vi "Dual_PID_tester.vi"() -> ()   [LabVIEW 2013]
uses:
  DataMode.ctl
  Input_5782/5782_states.ctl
  <vilib>/Platform/TimedLoop/XDataNode/timing_clust.ctl
  <vilib>/Platform/TimedLoop/XDataNode/nitl_modes.ctl
  <vilib>/Platform/TimedLoop/XDataNode/wakeup.ctl
  <vilib>/rvi/FXPMathLib/FxpConvert/subVIs/nifxpmath_Convert_SimConfig.ctl
  <vilib>/fxp/LVFixedPointQuantizationPolicyTypeDef.ctl
  <vilib>/fxp/LVFixedPointOverflowPolicyTypeDef.ctl
  <vilib>/rvi/Emulation/niFpgaSctlEmulationGetInTimedLoop.vi
  <vilib>/rvi/Emulation/niFpgaEmulationReportErrorSimple.vi
  <vilib>/rvi/Emulation/niFpgaGetClockAttributes.vi
  <vilib>/rvi/eio/common/nirviEmuTemplateMethod_errors.vi
  <vilib>/rvi/Emulation/niFpgaCriticalErrorInLSC.vi
  <vilib>/rvi/FXPMathLib/FxpConvert/simVIs/DllFxpConvertTemp_sub.vi
  <vilib>/rvi/FIFO/Fifo_Resource/nirvififoEmulationWriteFpgaImpl.vi
  <vilib>/rvi/DataTransferAndStorage/Container/Common/niFpgaContainerGetUniqueNameForEmu.vi
  <vilib>/rvi/DataTransferAndStorage/Register/Emulation/niFpgaRegisterEmulationFpgaImpl.vi
  <instcachedir>/0/niFpgaRegisterEmulationFpgaImpl_DCF4BC0110594B98B44A971D60CEEC4D.lvgen/niFpgaRegisterEmulationFpgaImpl_DCF4BC0110594B98B44A971D60CEEC4D_011.vi
  <instcachedir>/0/niFpgaRegisterEmulationFpgaImpl_DCF4BC0110594B98B44A971D60CEEC4D.lvgen/niFpgaRegisterEmulationFpgaImpl_DCF4BC0110594B98B44A971D60CEEC4D_012.vi
  <instcachedir>/0/niFpgaRegisterEmulationFpgaImpl_DCF4BC0110594B98B44A971D60CEEC4D.lvgen/niFpgaRegisterEmulationFpgaImpl_DCF4BC0110594B98B44A971D60CEEC4D_003.vi
  <instcachedir>/0/niFpgaRegisterEmulationFpgaImpl_DCF4BC0110594B98B44A971D60CEEC4D.lvgen/niFpgaRegisterEmulationFpgaImpl_DCF4BC0110594B98B44A971D60CEEC4D_007.vi
  <instcachedir>/0/niFpgaRegisterEmulationFpgaImpl_DCF4BC0110594B98B44A971D60CEEC4D.lvgen/niFpgaRegisterEmulationFpgaImpl_DCF4BC0110594B98B44A971D60CEEC4D_008.vi
  <instcachedir>/0/niFpgaRegisterEmulationFpgaImpl_DCF4BC0110594B98B44A971D60CEEC4D.lvgen/niFpgaRegisterEmulationFpgaImpl_DCF4BC0110594B98B44A971D60CEEC4D_021.vi
  <instcachedir>/0/niFpgaRegisterEmulationFpgaImpl_DCF4BC0110594B98B44A971D60CEEC4D.lvgen/niFpgaRegisterEmulationFpgaImpl_DCF4BC0110594B98B44A971D60CEEC4D_020.vi
  <instcachedir>/0/niFpgaRegisterEmulationFpgaImpl_DCF4BC0110594B98B44A971D60CEEC4D.lvgen/niFpgaRegisterEmulationFpgaImpl_DCF4BC0110594B98B44A971D60CEEC4D_009.vi
  <vilib>/rvi/FIFO/Fifo_Resource/nirvififoEmulationReadFpgaImpl.vi
  <vilib>/rvi/interface/RandomDataEmulation/nirviRandomDataMultiElementFPGAFIFO.vi
  <instcachedir>/0/nirviRandomDataMultiElementFPGAFIFO_F2B80EDE0D7944A08478D8D26097D4DB.lvgen/nirviRandomDataMultiElementFPGAFIFO_F2B80EDE0D7944A08478D8D26097D4DB_005.vi
  <vilib>/rvi/interface/RandomDataEmulation/niFpgaRandomDataHandleErrors.vi
  <instcachedir>/0/niFpgaRegisterEmulationFpgaImpl_DCF4BC0110594B98B44A971D60CEEC4D.lvgen/niFpgaRegisterEmulationFpgaImpl_DCF4BC0110594B98B44A971D60CEEC4D_013.vi
  <vilib>/rvi/interface/RandomDataEmulation/nirviRandomDataFPGAFIFO.vi
  <vilib>/Platform/TimedLoop/XDataNode/XDataNode.xnode
  <vilib>/eio/EIONode/EIONode.xnode
  <vilib>/rvi/FXPMathLib/FxpInterpret/XNode/nifxpmath_Interpret.xnode
  <vilib>/rvi/FXPMathLib/FxpConvert/XNode/nifxpmath_Convert.xnode
  <vilib>/rvi/DataTransferAndStorage/Container/XNode/niFpgaContainer.xnode
  <vilib>/rvi/FIFO/Fifo_Resource/nirvififoEmulationWrite.vi
  <vilib>/rvi/FXPMathLib/FxpSub/XNode/nifxpmath_Sub.xnode
  <vilib>/rvi/DataTransferAndStorage/Register/Emulation/niFpgaRegisterEmulation.vi
  <vilib>/rvi/FIFO/Fifo_Resource/nirvififoEmulationRead.vi
  <vilib>/rvi/interface/RandomDataEmulation/nirviRandomDataFpgaMultiElementTemplate.vi
  <vilib>/rvi/interface/RandomDataEmulation/nirviRandomDataFpgaReadWriteTemplate.vi
  <vilib>/Platform/TimedLoop/XDataNode/XDNodeRunTimeDep.lvlib
  <vilib>/rvi/FXPMathLib/sim/FxpSim.dll
panel:
  in  "delay phase":fxp<+,64,64>
  in  "5782 record length":u16=4000 caption="Samples Per Trigger" min=1 step=1
  in  "Trigger Acquisition":bool
  in  "5782 record length":u16=4000 caption="Samples Per Trigger" min=1 step=1
  in  "Trigger Acquisition":bool
  in  "AM phase":fxp<+,64,64>
  in  "Continuous":bool
  in  "Downsample":fxp<+,8,8>=1.0
  in  "new coeffs":bool
  in  "FIR coeffs":fxp<+/-,18,18>[](array[numeric])
  in  "CIC Gain":fxp<+/-,32,1>=0.00390625 format="%#_32g"
  in  "Acquisition running":bool
  in  "Phase output":fxp<+,64,64>[](array[numeric])=[0.0, 0.0, 0.0, 0.0, 0.0, 0.0, 0.0, 0.0]
  in  "Simulated phase 5782":fxp<+,64,64>[](array[numeric])=[0.0, 0.0]
  in  "Mode":T1
  in  "Phase 5782":fxp<+,64,64>[](array[numeric])=[0.0, 0.0]
  out "IO Module\\Trigger Input":bool
  in  "IO Module\\AO Data Sync":bool=TRUE
  in  "IO Module\\SPI Write Data":u16
  out "IO Module\\SPI Read Data":u8
  in  "IO Module\\SPI Read":bool
  in  "IO Module\\SPI Write":bool
  in  "IO Module\\SPI Address":u16
  in  "IO Module\\SPI Device":u8
  out "IO Module\\SPI Idle":bool
  in  "User Command Commit":bool
  in  "User Command":u8
  out "User Command Idle":bool
  out "User Command Status":u8
  in  "User Data 0":u8
  in  "User Data 1":u8
  out "PLL Locked":bool
  out "User Error":bool
  out "Configured?":bool
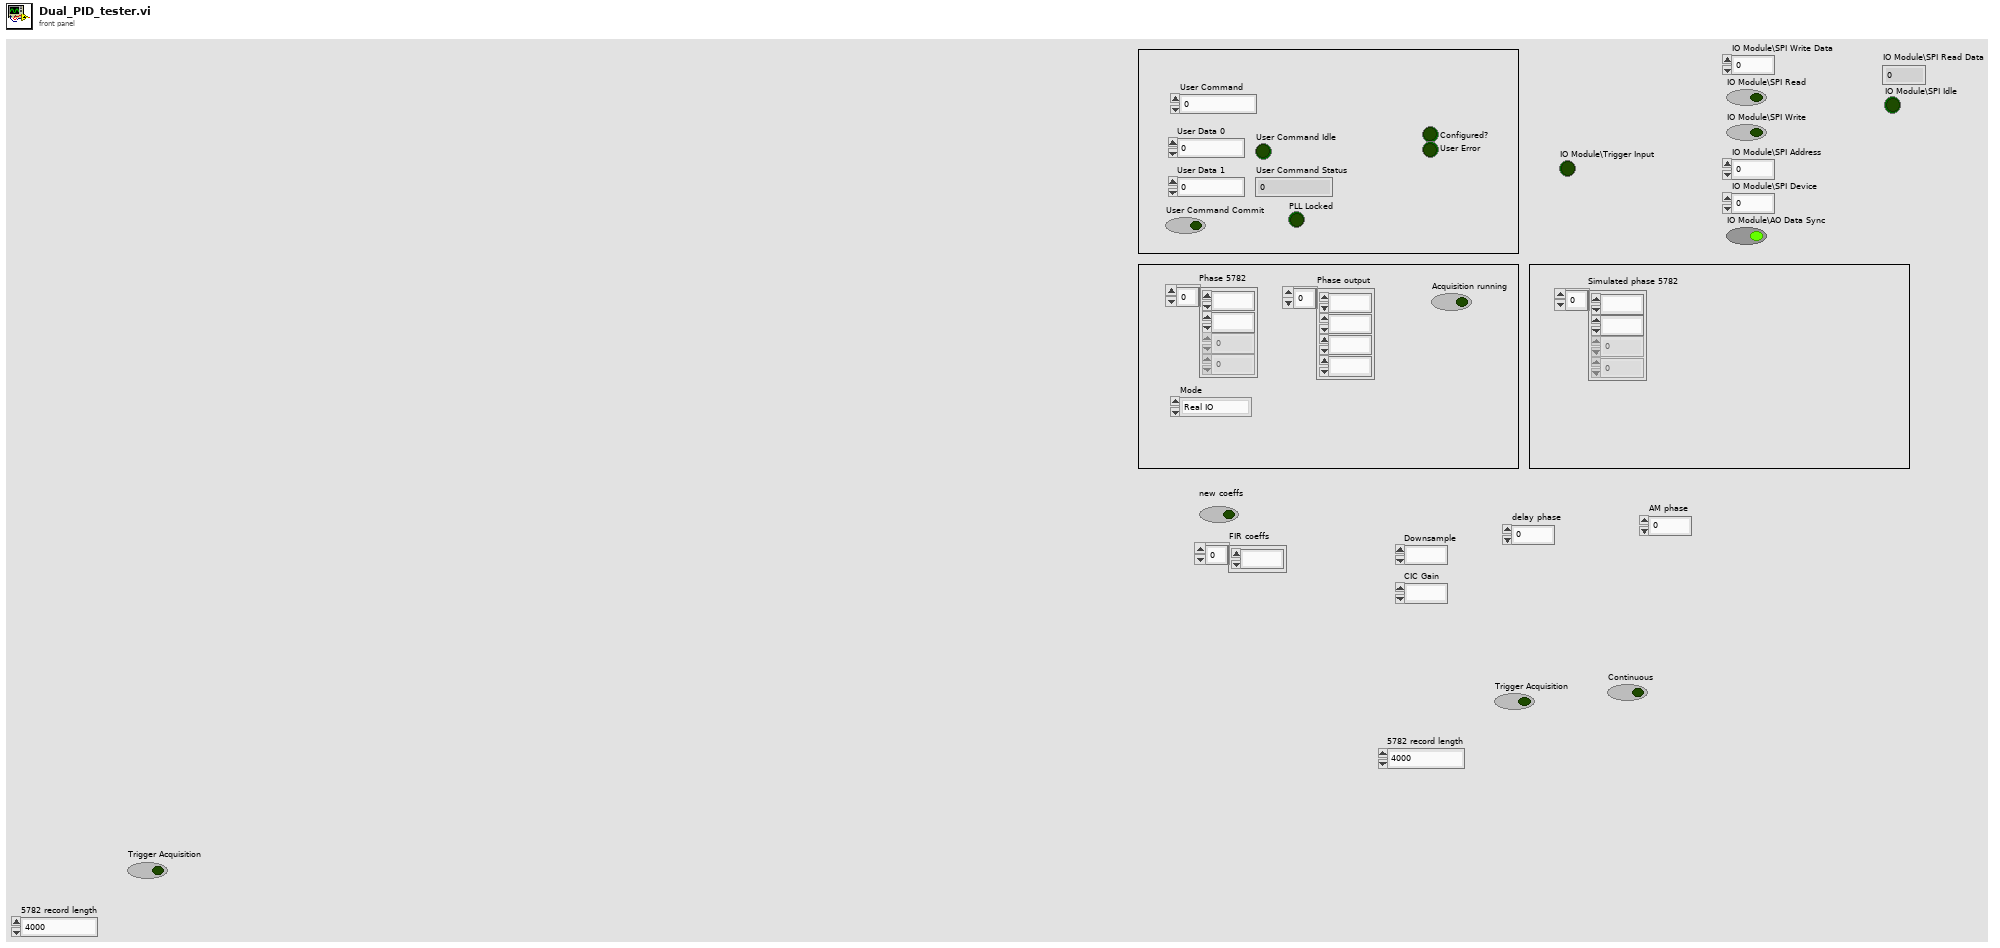
[diagram p1: front panel]
types:
  T1 = typedef "DataMode.ctl" = enum16{"Real IO", "Simulated"}
  T2 = typedef "5782_states.ctl" = enum8{"Wait for trigger", "Acquisition", "Send record length", "Quiet period"}
  T3 = typedef "XDNodeRunTimeDep.lvlib/timing_clust.ctl" = cluster{"Expected End [f-1]":u64, "Actual End [f-1]":u64, "Finished Late? [f-1]":bool, "Expected End [i-1]":u64, "Actual End [i-1]":u64, "Finished Late? [i-1]":bool, "Expected Start [i]":u64, "Actual Start [i]":u64, "Expected Start [f]":u64, "Actual Start [f]":u64, "Source Name":string, "Structure Name":string, "Period":i64, "Deadline":i64, "Offset":i64, "Start":i64, "Priority":i32, "Timeout":i32, "Mode":T4, "Wakeup Reason":T5, "Error":errorcluster, "Source Type":string, "Secondary Source Type":string, "Global End Time":u64, "Global Start Time":u64, "Frame Duration":u64, "Iteration Duration":u64, "Assigned CPU":i32, "I/O Scan Engine Mode":u32}
  T4 = typedef "XDNodeRunTimeDep.lvlib/nitl_modes.ctl" = enum32{"No Change", "Process missed periods, maintain original phase", "Discard missed periods, maintain original phase", "Process missed periods, ignore original phase", "Discard missed periods, ignore original phase"}
  T5 = typedef "XDNodeRunTimeDep.lvlib/wakeup.ctl" = enum32{"Normal", "Aborted", "Asynchronous wakeup", "Timing source error", "Timed loop error", "Timeout"}
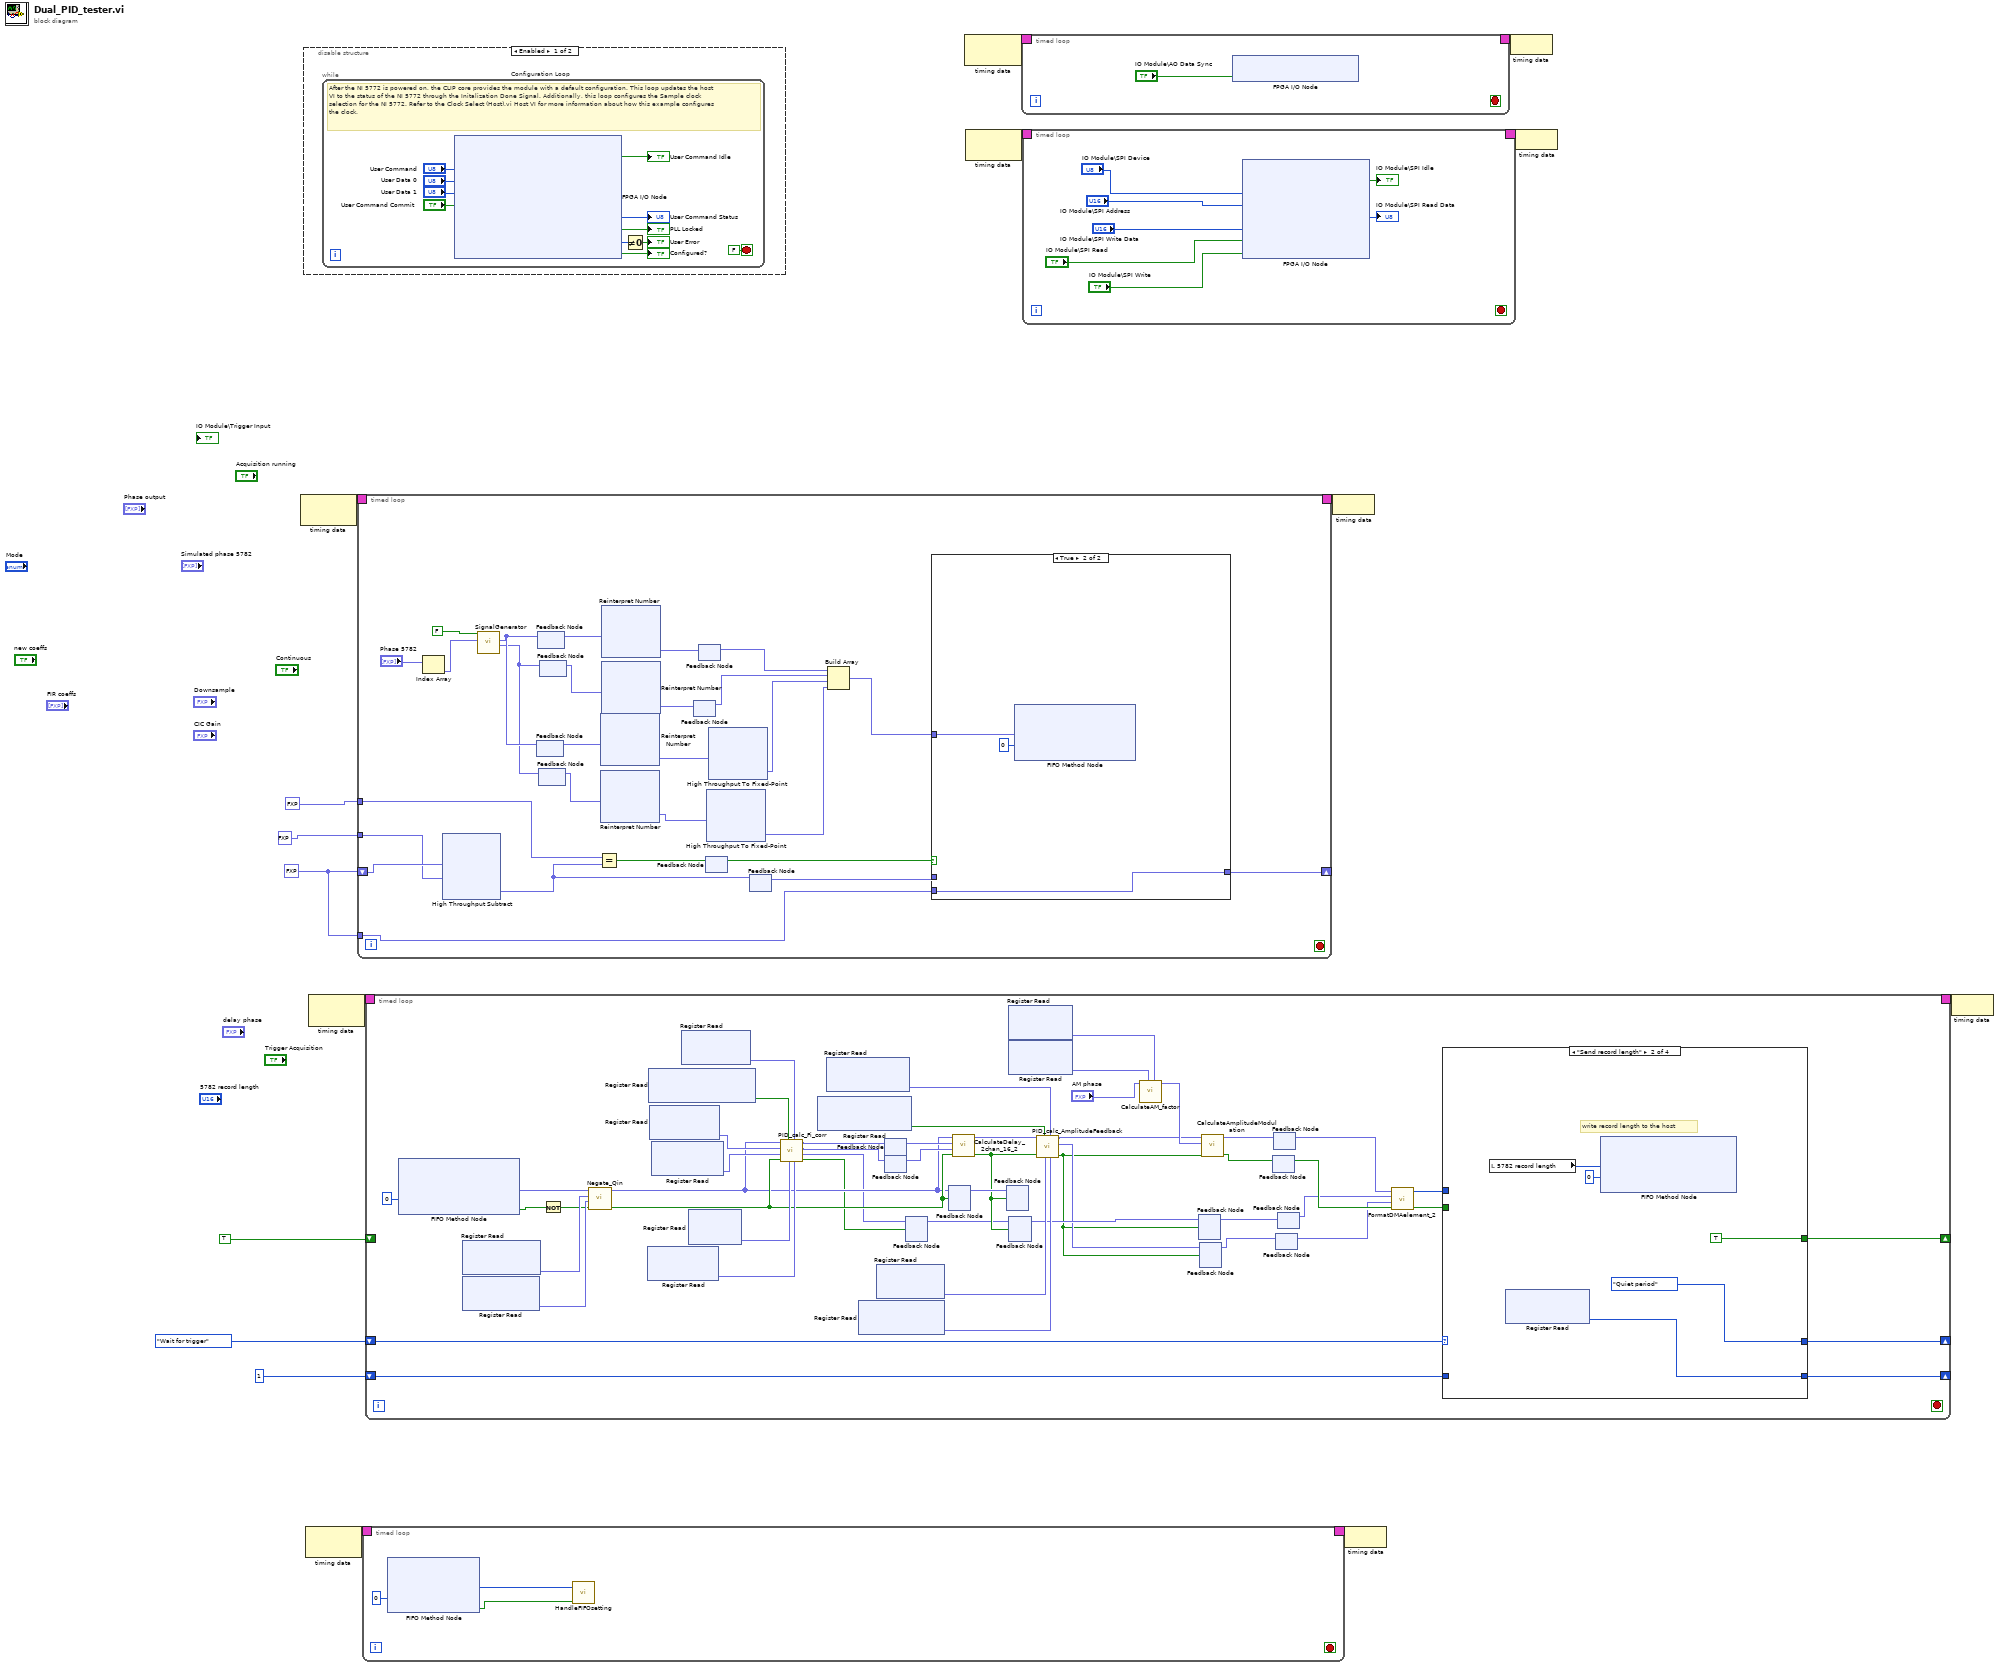
[diagram p0: block diagram]
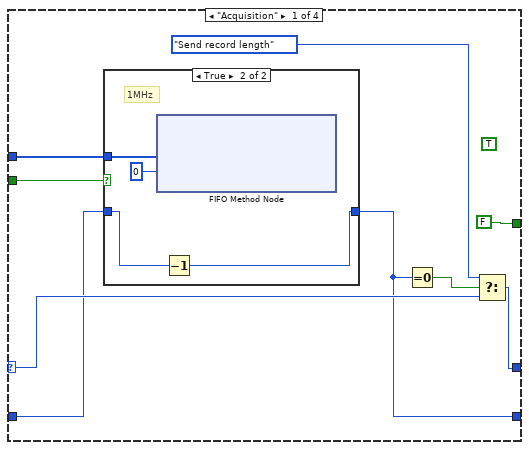
[diagram p2: hidden frame]
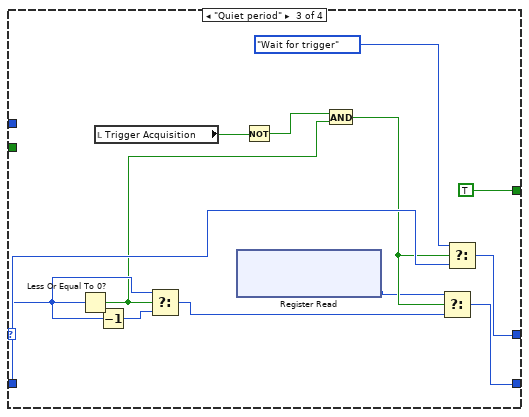
[diagram p4: hidden frame]
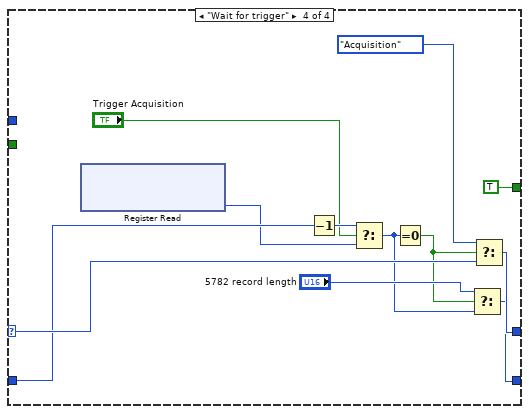
[diagram p5: hidden frame]
diagram:
  w8 = fxp<+/-,8,8> 5.0 ("x")
  n1 = node-c288() -> (w7:T3)  [unwired: 1 in]
  n2 = disable-structure shown="Enabled" {
    frame Enabled {
      n3 = while "Configuration Loop" {
        stop <- FALSE stop-if-true
        # "After the NI 5772 is powered on, the CLIP core provides the module with a default configuration. This loop updates the host VI to the status of the NI 5772 through the Initalization Done Signal. Additionally, this loop configures the Sample clock selection for the NI 5772. Refer to the Clock Select (Host).vi Host VI for more information about how this example configures the clock."
        n4 = xnode "FPGA I/O Node"("IO Module\\User Command"="User Command", "IO Module\\User Data 0"="User Data 0", "IO Module\\User Data 1"="User Data 1", "IO Module\\User Command Commit"="User Command Commit") -> ("IO Module\\User Command Idle"=→"User Command Idle":bool, "IO Module\\User Command Status"=→"User Command Status":u8, "IO Module\\PLL Locked"=→"PLL Locked":bool, "IO Module\\User Error"=w22:u8, "IO Module\\Initialization Done"=→"Configured?":bool)  [unwired: 9 in, 9 out]
        n5 = Not Equal To 0?(x=w22) -> (x != 0?=→"User Error":bool)
      }
    }
    frame Disabled {
    }
  }
  n6 = node-c288() -> (w16:T3)  [unwired: 1 in]
  n7 = node-c288() -> (w5:T3)  [unwired: 1 in]
  n8 = timed-loop {
    shift-right: [w50] -> _
    shift-left: w8 -> [w54]
    tunnel: fxp<+/-,8,8> 1.0 ("y") -> [w53]
    tunnel: fxp<+/-,8,8> 0.0 ("y") -> [w52]
    tunnel: w8 -> [w51]
    timing: w7 -> [_]
    timing-out: [_] -> w6
    stop <- _ stop-if-true
    n9 = Index Array(array="Phase 5782") -> (element=w28:fxp<+,64,64>)  [unwired: 1 in]
    n10 = xnode "High Throughput Subtract"("x"=w54, "y"=w53) -> ("x-y"=w47:fxp<+/-,8,8>)
    n11 = call "SignalGenerator.vi"("phase"=w28, "Reset"=FALSE) -> ("Cos"=w39:fxp<+/-,16,0>, "Sin"=w40:fxp<+/-,16,0>)  [unwired: 7 in, 1 out]
    n12 = feedback #1() -> (w41:fxp<+/-,16,0>)  [unwired: 1 in]
    n13 = feedback-in #1(w40) -> ()
    n14 = feedback #2() -> (w44:fxp<+/-,16,0>)  [unwired: 1 in]
    n15 = feedback-in #2(w40) -> ()
    n16 = feedback #3() -> (w42:fxp<+/-,16,0>)  [unwired: 1 in]
    n17 = feedback-in #3(w39) -> ()
    n18 = feedback #4() -> (w43:fxp<+/-,16,0>)  [unwired: 1 in]
    n19 = feedback-in #4(w39) -> ()
    n20 = Equal?(x=w52, y=w47) -> (x = y?=w49:bool)
    n21 = xnode "Reinterpret Number"("x"=w41) -> ("y"=w38:fxp<+/-,16,15>)
    n22 = xnode "Reinterpret Number"("x"=w42) -> ("y"=w37:fxp<+/-,16,15>)
    n23 = xnode "Reinterpret Number"("x"=w44) -> ("y"=w36:fxp<+/-,16,14>)
    n24 = xnode "Reinterpret Number"("x"=w43) -> ("y"=w35:fxp<+/-,16,14>)
    n25 = feedback #5() -> (w33:fxp<+/-,16,14>)  [unwired: 1 in]
    n26 = feedback-in #5(w35) -> ()
    n27 = feedback #6() -> (w34:fxp<+/-,16,14>)  [unwired: 1 in]
    n28 = feedback-in #6(w36) -> ()
    n29 = feedback #7() -> (w48:bool)  [unwired: 1 in]
    n30 = feedback-in #7(w49) -> ()
    n31 = xnode "High Throughput To Fixed-Point"("x"=w37) -> ("y"=w31:fxp<+/-,16,14>)
    n32 = xnode "High Throughput To Fixed-Point"("x"=w38) -> ("y"=w32:fxp<+/-,16,14>)
    n33 = feedback #8() -> (w46:fxp<+/-,8,8>)  [unwired: 1 in]
    n34 = feedback-in #8(w47) -> ()
    n35 = Build Array(w34, w33, w32, w31) -> (w30:fxp<+/-,16,14>[])
    n36 = case shown="True" w48 {
      tunnel: w51 -> [_ w102]
      tunnel: w46 -> [w99 _]
      tunnel: [w99 w102] -> w50
      tunnel: w30 -> [_ w100]
      frame False {
      }
      frame True {
        n37 = xnode ("FIFO Method Node")("Element"=w100, "Timeout"=0) -> ()  [unwired: 1 in, 2 out]
      }
    }
  }
  n38 = timed-loop {
    timing: w16 -> [_]
    timing-out: [_] -> w15
    stop <- _ stop-if-true
    n39 = xnode ("FIFO Method Node")("Timeout"=0) -> ("Element"=w106:u64, "Timed Out?"=w105:bool)  [unwired: 1 in, 1 out]
    n40 = call "HandleFIFOsetting.vi"("timed out"=w105, "Value"=w106) -> ()  [unwired: 10 in]
  }
  n41 = timed-loop {
    timing: w5 -> [_]
    timing-out: [_] -> w4
    shift-right: [w158] -> _
    shift-left: 5782_states."Wait for trigger" ("5782 states") -> [w160]
    shift-right: [w157] -> _
    shift-left: u16 1 ("trigger samples") -> [w159]
    shift-right: [w152] -> _
    shift-left: TRUE -> [_]
    stop <- _ stop-if-true
    n42 = xnode ("FIFO Method Node")("Timeout"=0) -> ("Element"=w141:fxp<+/-,16,14>[], "Timed Out?"=w155:bool)  [unwired: 1 in, 1 out]
    n43 = xnode ("Register Read")() -> ("Data"=w148:fxp<+/-,16,14>)  [unwired: 1 in, 1 out]
    n44 = xnode ("Register Read")() -> ("Data"=w149:fxp<+/-,16,14>)  [unwired: 1 in, 1 out]
    n45 = Not(x=w155) -> (.not. x?=w142:bool)
    n46 = call "Negate_Qin.vi"("valid in"=w142, "DC offset chan 1"=w148, "DC offset chan 0"=w149, "Data in"=w141) -> ("valid out"=w132:bool, "Data out"=w131:fxp<+/-,16,14>[])  [unwired: 6 in]
    n47 = xnode ("Register Read")() -> ("Data"=w139:fxp<+/-,32,4>)  [unwired: 1 in, 1 out]
    n48 = xnode ("Register Read")() -> ("Data"=w136:bool)  [unwired: 1 in, 1 out]
    n49 = xnode ("Register Read")() -> ("Data"=w137:fxp<+/-,32,4>)  [unwired: 1 in, 1 out]
    n50 = xnode ("Register Read")() -> ("Data"=w138:fxp<+/-,32,4>)  [unwired: 1 in, 1 out]
    n51 = xnode ("Register Read")() -> ("Data"=w135:fxp<+/-,32,4>)  [unwired: 1 in, 1 out]
    n52 = xnode ("Register Read")() -> ("Data"=w140:fxp<+/-,32,4>)  [unwired: 1 in, 1 out]
    n53 = call "PID_calc_Fi_corr.vi"("Kd/Tau"=w139, "Ki*Tau"=w135, "Kp"=w140, "Enabled"=w136, "input valid"=w132, "Fi_delta"=w138, "Fi_start"=w137, "Data in"=w131) -> ("output valid"=w129:bool, "c out"=w130:fxp<+/-,32,4>, "cos_fi_korr"=w133:fxp<+/-,16,2>, "sin fi_korr"=w134:fxp<+/-,16,2>)
    n54 = xnode ("Register Read")() -> ("Data"=w146:bool)  [unwired: 1 in, 1 out]
    n55 = xnode ("Register Read")() -> ("Data"=w143:fxp<+/-,32,6>)  [unwired: 1 in, 1 out]
    n56 = xnode ("Register Read")() -> ("Data"=w144:fxp<+/-,32,6>)  [unwired: 1 in, 1 out]
    n57 = xnode ("Register Read")() -> ("Data"=w145:fxp<+/-,32,6>)  [unwired: 1 in, 1 out]
    n58 = feedback-in #9(w134) -> ()
    n59 = feedback #9() -> (w151:fxp<+/-,16,2>)  [unwired: 1 in]
    n60 = feedback #10() -> (w150:fxp<+/-,16,2>)  [unwired: 1 in]
    n61 = feedback-in #10(w133) -> ()
    n62 = feedback #11() -> (w126:fxp<+/-,32,4>)  [unwired: 1 in]
    n63 = feedback-in #11(w130, w129) -> ()
    n64 = feedback #12() -> (w128:fxp<+/-,16,14>[])  [unwired: 1 in]
    n65 = feedback-in #12(w131, w132) -> ()
    n66 = call "CalculateDelay_2chan_16_2.vi"("input valid"=w132, "cos_fi"=w150, "sin fi"=w151, "Data in"=w131) -> ("output valid"=w127:bool, "Data out"=w147:fxp<+/-,16,14>[])  [unwired: 6 in]
    n67 = feedback #13() -> ()  [unwired: 2 in]
    n68 = feedback-in #13(w128, w127) -> ()
    n69 = xnode ("Register Read")() -> ("Data"=w123:fxp<+/-,16,2>)  [unwired: 1 in, 1 out]
    n70 = xnode ("Register Read")() -> ("Data"=w124:fxp<+/-,16,2>)  [unwired: 1 in, 1 out]
    n71 = feedback #14() -> (w125:fxp<+/-,32,4>)  [unwired: 1 in]
    n72 = feedback-in #14(w126, w127) -> ()
    n73 = call "PID_calc_AmplitudeFeedback.vi"("Kd/Tau"=w144, "Ki*Tau"=w143, "Kp"=w145, "Enabled"=w146, "input valid"=w127, "Data in"=w147) -> ("output valid"=w114:bool, "c(t)"=w115:fxp<+/-,32,21>, "data out"=w120:fxp<+/-,16,14>[])  [unwired: 2 in, 1 out]
    n74 = call "CalculateAM_factor.vi"("b_am"=w123, "a_am"=w124, "AM phase"="AM phase") -> ("AM_factor"=w122:fxp<+/-,16,2>)  [unwired: 7 in, 1 out]
    n75 = feedback #15() -> (w113:fxp<+/-,32,4>)  [unwired: 1 in]
    n76 = feedback-in #15(w125, w114) -> ()
    n77 = feedback #16() -> (w112:fxp<+/-,32,21>)  [unwired: 1 in]
    n78 = feedback-in #16(w115, w114) -> ()
    n79 = call "CalculateAmplitudeModulation.vi"("input valid"=w114, "AM_factor"=w122, "Data in"=w120) -> ("output valid"=w118:bool, "Data out"=w119:fxp<+/-,16,14>[])  [unwired: 7 in]
    n80 = feedback #17() -> (w117:bool)  [unwired: 1 in]
    n81 = feedback-in #17(w118) -> ()
    n82 = feedback #18() -> (w116:fxp<+/-,16,14>[])  [unwired: 1 in]
    n83 = feedback-in #18(w119) -> ()
    n84 = feedback #19() -> (w110:fxp<+/-,32,21>)  [unwired: 1 in]
    n85 = feedback-in #19(w112) -> ()
    n86 = feedback #20() -> (w111:fxp<+/-,32,4>)  [unwired: 1 in]
    n87 = feedback-in #20(w113) -> ()
    n88 = call "FormatDMAelement_2.vi"("valid in"=w117, "c(t) - AM"=w110, "c(t) - Phase"=w111, "Data in"=w116) -> ("valid out"=w153:bool, "Element"=w154:u64[])  [unwired: 6 in]
    n89 = case shown="\"Send record length\"" w160 {
      selector: w160 -> [w169 _ w191 w204]
      tunnel: w159 -> [w165 _ w184 w195]
      tunnel: [w168 5782_states."Quiet period" ("5782 states") w190 w203] -> w158
      tunnel: [w162 w175 w192 w202] -> w157
      tunnel: w154 -> [w163 _ _ _]
      tunnel: w153 -> [w164 _ _ _]
      tunnel: [FALSE TRUE TRUE TRUE] -> w152
      frame "Acquisition" {
        (unwired) TRUE
        n90 = case shown="True" w164 {
          tunnel: w163 -> [_ w174]
          tunnel: [w170 w171] -> w162
          tunnel: w165 -> [w170 w172]
          frame False {
          }
          frame True {
            # "1MHz"
            n91 = xnode ("FIFO Method Node")("Element"=w174, "Timeout"=0) -> ()  [unwired: 1 in, 2 out]
            n92 = Decrement(x=w172) -> (x-1=w171:u16)
          }
        }
        n93 = Equal To 0?(x=w162) -> (x = 0?=w166:bool)
        n94 = Select(t=5782_states."Send record length" ("5782 states"), s=w166, f=w169) -> (s? t:f=w168:T2)
      }
      frame "Send record length" {
        # "write record length to the host"
        n95 = local read "5782 record length"() -> (w176:u16)
        n96 = xnode ("Register Read")() -> ("Data"=w175:u16)  [unwired: 1 in, 1 out]
        n97 = xnode ("FIFO Method Node")("Element"=w176, "Timeout"=0) -> ()  [unwired: 1 in, 2 out]
      }
      frame "Quiet period" {
        n98 = Less Or Equal To 0?(x=w184) -> (x <= 0?=w183:bool)
        n99 = local read "Trigger Acquisition"() -> (w187:bool)
        n100 = Decrement(x=w184) -> (x-1=w185:u16)
        n101 = Select(t=w184, s=w183, f=w185) -> (s? t:f=w182:u16)
        n102 = xnode ("Register Read")() -> ("Data"=w181:u16)  [unwired: 1 in, 1 out]
        n103 = Not(x=w187) -> (.not. x?=w180:bool)
        n104 = And(x=w180, y=w183) -> (x .and. y?=w189:bool)
        n105 = Select(t=w181, s=w189, f=w182) -> (s? t:f=w192:u16)
        n106 = Select(t=5782_states."Wait for trigger" ("5782 states"), s=w189, f=w191) -> (s? t:f=w190:T2)
      }
      frame "Wait for trigger" {
        n107 = xnode ("Register Read")() -> ("Data"=w194:u16)  [unwired: 1 in, 1 out]
        n108 = Decrement(x=w195) -> (x-1=w196:u16)
        n109 = Select(t=w196, s="Trigger Acquisition", f=w194) -> (s? t:f=w197:u16)
        n110 = Equal To 0?(x=w197) -> (x = 0?=w198:bool)
        n111 = Select(t="5782 record length", s=w198, f=w197) -> (s? t:f=w202:u16)
        n112 = Select(t=5782_states."Acquisition" ("5782 states"), s=w198, f=w204) -> (s? t:f=w203:T2)
      }
    }
  }
  n113 = node-c288() -> (w12:T3)  [unwired: 1 in]
  n114 = node-c288() -> (w14:T3)  [unwired: 1 in]
  n115 = timed-loop {
    timing: w12 -> [_]
    timing-out: [_] -> w11
    stop <- _ stop-if-true
    n116 = xnode "FPGA I/O Node"("IO Module\\AO Data Sync"="IO Module\\AO Data Sync") -> ()  [unwired: 1 in, 1 out]
  }
  n117 = timed-loop {
    timing: w14 -> [_]
    timing-out: [_] -> w13
    stop <- _ stop-if-true
    n118 = xnode "FPGA I/O Node"("IO Module\\SPI Device"="IO Module\\SPI Device", "IO Module\\SPI Address"="IO Module\\SPI Address", "IO Module\\SPI Write Data"="IO Module\\SPI Write Data", "IO Module\\SPI Read"="IO Module\\SPI Read", "IO Module\\SPI Write"="IO Module\\SPI Write") -> ("IO Module\\SPI Idle"=→"IO Module\\SPI Idle":bool, "IO Module\\SPI Read Data"=→"IO Module\\SPI Read Data":u8)  [unwired: 7 in, 7 out]
  }
  n119 = node-c288(w6) -> ()
  n120 = node-c288(w15) -> ()
  n121 = node-c288(w11) -> ()
  n122 = node-c288(w13) -> ()
  n123 = node-c288(w4) -> ()
